vi "簇与数组转换.vi"() -> ()   [LabVIEW 2010]
panel:
  out "数组":i32[](array[numeric])
  out "簇":T1
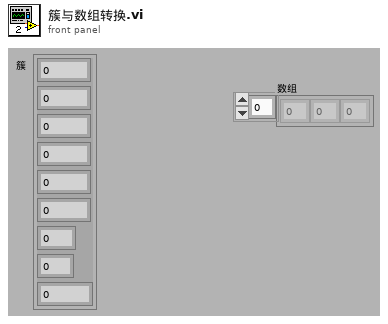
[diagram p1: front panel]
types:
  T1 = cluster{i32, i32, i32, i32, i32, i32, i32, i32, i32}
  T2 = cluster{"[0]":i32, "[1]":i32, "[2]":i32, "[3]":i32, "[4]":i32, "[5]":i32, "[6]":i32, "[7]":i32, "[8]":i32}
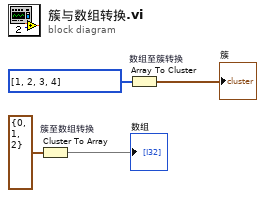
[diagram p0: block diagram]
diagram:
  n1 = Cluster To Array "簇至数组转换"(cluster=cluster{i32, i32, i32} {0, 1, 2}) -> (array=→"数组":i32[])
  n2 = Array To Cluster "数组至簇转换"(array=i32[] [1, 2, 3, 4]) -> (cluster=→"簇":T2)
